vi "1DGaussian001.vi"(1 "Parameters":dbl[](array[numeric]) format="%.2f") -> (0 "Gaussian":dbl[](array[numeric]) format="%.2f")   [LabVIEW 2016]
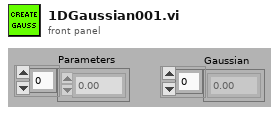
[diagram p1: front panel]
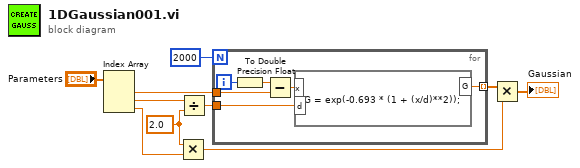
[diagram p0: block diagram]
diagram:
  w1 = 2.0 ("y")
  n1 = Index Array(array="Parameters") -> (element #1=w3:dbl, element #2=w10:dbl, element #3=w5:dbl)  [unwired: 3 in]
  n2 = Multiply(x=w1, y=w5) -> (x*y=w2:dbl)
  n3 = Divide(x=w10, y=w1) -> (x/y=w8:dbl)
  n4 = for {
    N: 2000 ("samples") -> [_]
    tunnel: [w16] -> w7 mode=indexing
    tunnel: w8 -> [w15]
    tunnel: w3 -> [w14]
    i -> [w11]
    n5 = To Double Precision Float(number=w11) -> (double precision float=w12:dbl)
    n6 = Subtract(x=w12, y=w14) -> (x-y=w13:dbl)
    n7 = formula code="G = exp(-0.693 * (1 + (x/d)**2));"("x"=w13, "d"=w15) -> ("G"=w16:dbl)
  }
  n8 = Multiply(x=w7, y=w2) -> (x*y=→"Gaussian":dbl[])
